vi "Insert_Fix Node Terminals.vi"(6 "Inserted Node":refnum<vi>, 8 "error in (no error)":errorcluster, 9 "Original Wire":refnum<vi>, 11 "Node Name":string) -> (0 "error out":errorcluster)   [LabVIEW 2020]
doc: "When the LabVIEW Insert algorithm inserts the node in a non-ideal manner on a wire, this VI will fix the wiring in those specific cases."
uses:
  <vilib>/Utility/Data Type/Type Definitions/Data Type.ctl
  <vilib>/Utility/Data Type/NI_Data Type.lvlib
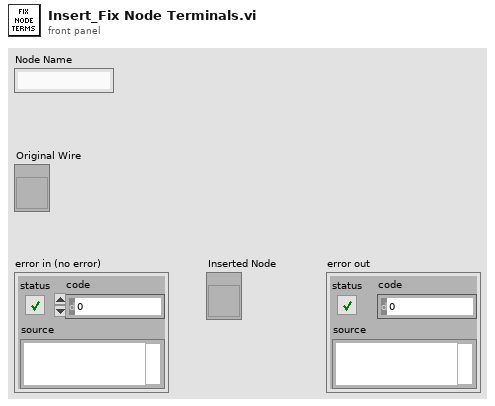
[diagram p1: front panel]
types:
  T1 = typedef "NI_Data Type.lvlib/Data Type.ctl" = enum8{"Invalid Type", "Void", "I8", "I16", "I32", "I64", "U8", "U16", "U32", "U64", "Single Float", "Double Float", "Extended Float", "Single Complex", "Double Complex", "Extended Complex", "Enum U8", "Enum U16", "Enum U32", "Enum U64", "Single Float With Unit", "Double Float With Unit", "Extended Float With Unit", "Single Complex with Unit", "Double Complex with Unit", "Extended Complex with Unit", "Boolean", "String", "Path", "Picture", "Tag", "Array", "Cluster", "Variant", "LV Variant", "Waveform", "Timestamp", "Digital Waveform", "Digital Data", "ExpressData", "Refnum", "External Data", "VI", "Poly VI", "LabVIEW Class Instance", "Fixed Point", "Set Collection", "Map Collection"}
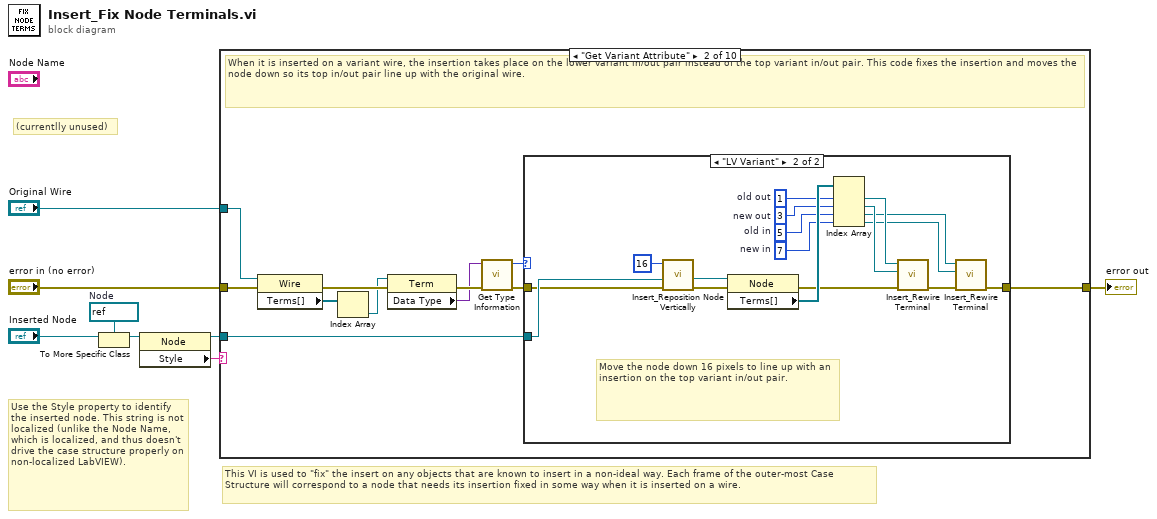
[diagram p0: block diagram]
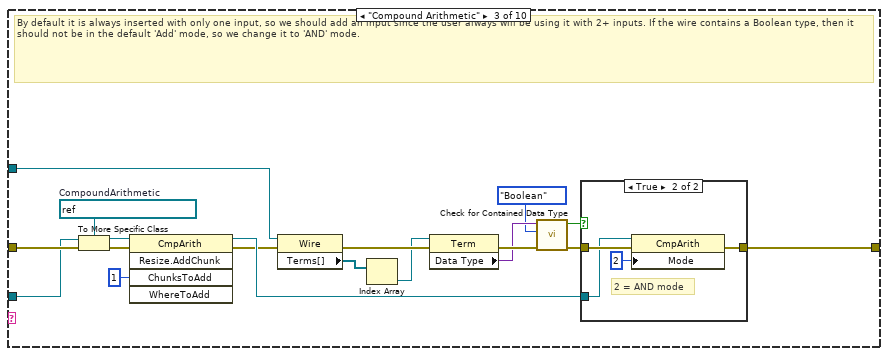
[diagram p4: hidden frame]
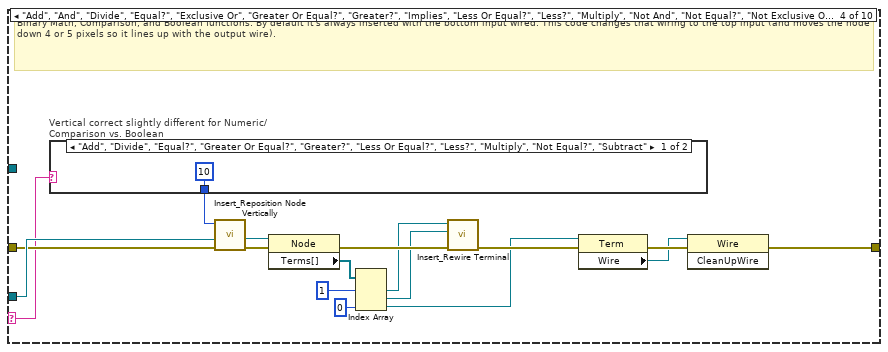
[diagram p6: hidden frame]
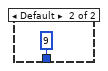
[diagram p7: hidden frame]
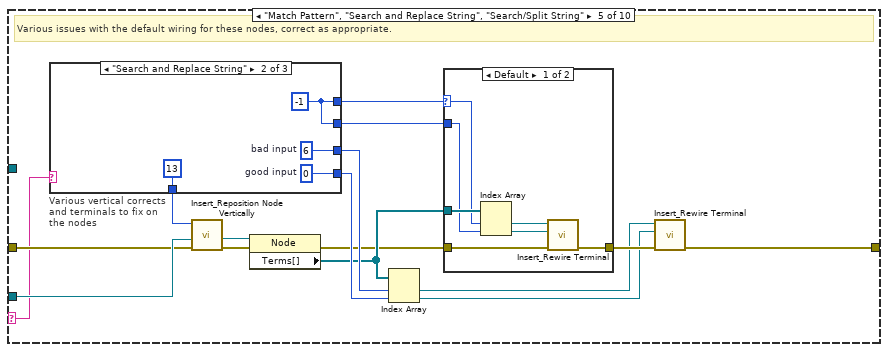
[diagram p8: hidden frame]
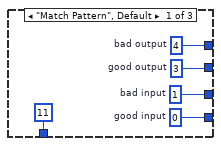
[diagram p10: hidden frame]
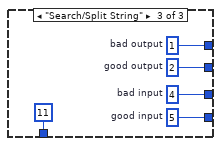
[diagram p11: hidden frame]
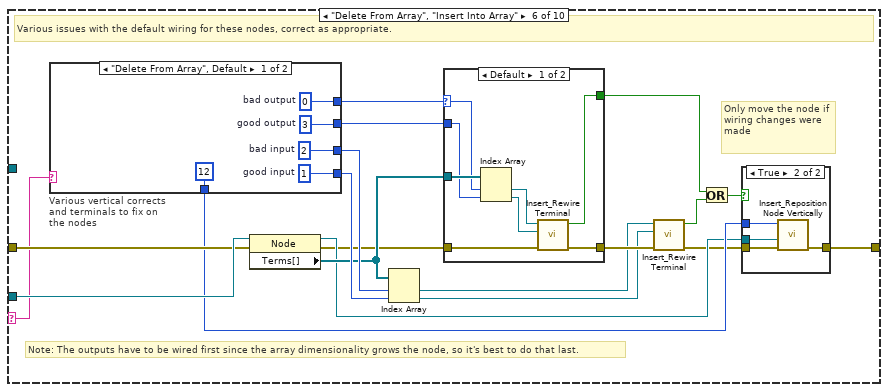
[diagram p12: hidden frame]
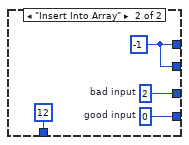
[diagram p15: hidden frame]
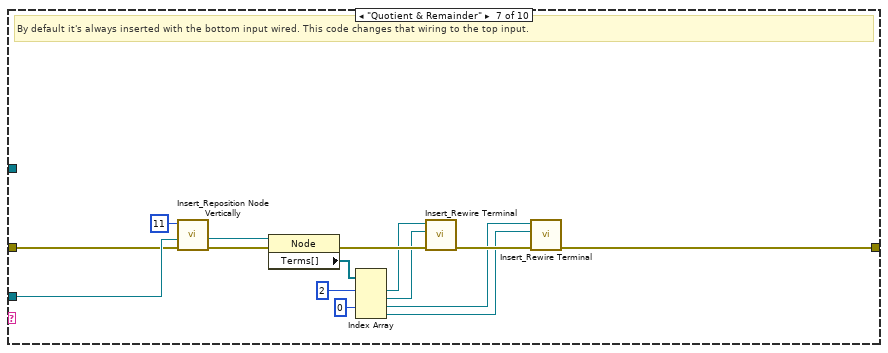
[diagram p16: hidden frame]
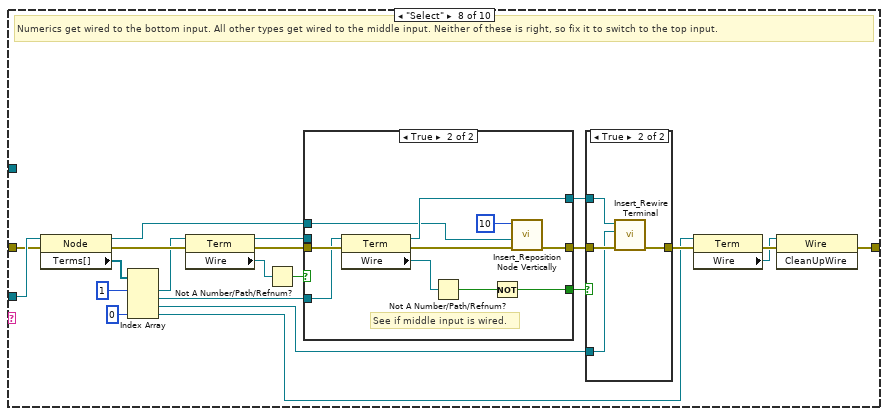
[diagram p17: hidden frame]
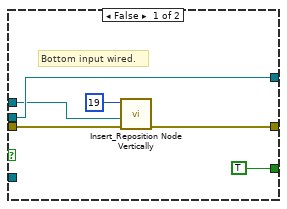
[diagram p19: hidden frame]
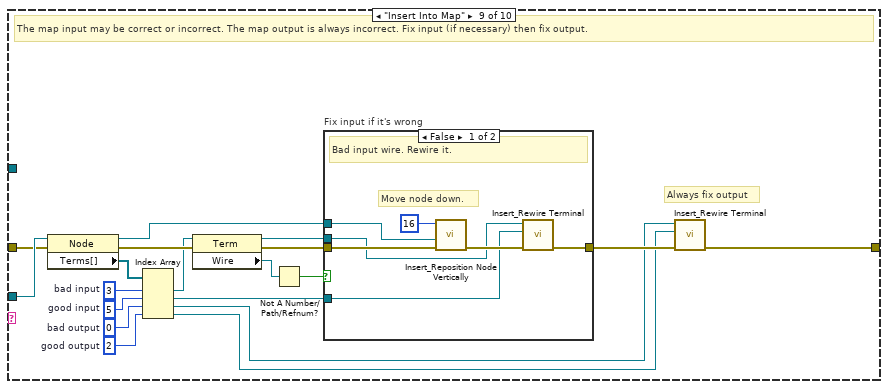
[diagram p20: hidden frame]
diagram:
  w3 = refnum<vi> refnum  # Node
  # "(currentlly unused)"
  # "Use the Style property to identify the inserted node. This string is not localized (unlike the Node Name, which is localized, and thus doesn't drive the case structure properly on non-localized LabVIEW)."
  # "This VI is used to \"fix\" the insert on any objects that are known to insert in a non-ideal way. Each frame of the outer-most Case Structure will correspond to a node that needs its insertion fixed in some way when it is inserted on a wire."
  n1 = To More Specific Class(target class=w3, reference="Inserted Node") -> (specific class reference=w4:refnum<vi>)  [unwired: 1 in, 1 out]
  n2 = property class="Node"(reference=w4) -> (reference out=w2:refnum<vi>, "Style"=w1:string)  [unwired: 1 in, 1 out]
  n3 = case shown="\"Get Variant Attribute\"" w1 {
    selector: w1 -> [_ _ _ w62 w81 w119 _ _ _ _]
    tunnel: "error in (no error)" -> [w9 w20 w44 w77 w95 w136 w174 w196 w236 w263]
    tunnel: [w9 w11 w49 w63 w84 w130 w167 w178 w223 w250] -> w6
    tunnel: "Original Wire" -> [_ w19 w56 _ _ _ _ _ _ _]
    tunnel: w2 -> [_ w10 w43 w78 w96 w137 w175 w197 w237 w264]
    frame Default {
      # "Not a Node that requires wire fixing."
    }
    frame "Get Variant Attribute" {
      # "When it is inserted on a variant wire, the insertion takes place on the lower variant in/out pair instead of the top variant in/out pair. This code fixes the insertion and moves the node down so its top in/out pair line up with the original wire."
      n4 = property class="Wire"(reference=w19, error in=w20) -> (error out=w17:errorcluster, "Terms[]"=w18:refnum<vi>[])  [unwired: 1 out]
      n5 = Index Array(array=w18) -> (element=w16:refnum<vi>)  [unwired: 1 in]
      n6 = property class="Term"(reference=w16, error in=w17) -> (error out=w15:errorcluster, "Data Type"=w14:variant)  [unwired: 1 out]
      n7 = call <vilib>:"Get Type Information.vi"("error in (no error)"=w15, "variant"=w14) -> ("error out"=w13:errorcluster, "type"=w12:T1)  [unwired: 5 in, 3 out]
      n8 = case shown="\"LV Variant\"" w12 {
        tunnel: w13 -> [w21 w37]
        tunnel: [w21 w24] -> w11
        tunnel: w10 -> [_ w38]
        frame Default {
          # "Do nothing if the insert took place on a non-variant wire, like the error cluster."
        }
        frame "LV Variant" {
          w32 = 7  # new in
          w33 = 5  # old in
          w34 = 3  # new out
          w35 = 1  # old out
          # "Move the node down 16 pixels to line up with an insertion on the top variant in/out pair."
          n9 = call <vilib>:"Insert_Reposition Node Vertically.vi"("error in"=w37, "Node in"=w38, "Vertical Change"=16 ("y")) -> ("error out"=w31:errorcluster, "Node out"=w23:refnum<vi>)  [unwired: 7 in]
          n10 = property class="Node"(reference=w23, error in=w31) -> (error out=w30:errorcluster, "Terms[]"=w36:refnum<vi>[])  [unwired: 1 out]
          n11 = Index Array(array=w36, index #1=w35, index #2=w34, index #3=w33, index #4=w32) -> (element #1=w29:refnum<vi>, element #2=w28:refnum<vi>, element #3=w26:refnum<vi>, element #4=w25:refnum<vi>)
          n12 = call <vilib>:"Insert_Rewire Terminal.vi"("error in"=w30, "New Terminal"=w28, "Old Terminal"=w29) -> ("error out"=w27:errorcluster)  [unwired: 7 in, 1 out]
          n13 = call <vilib>:"Insert_Rewire Terminal.vi"("error in"=w27, "New Terminal"=w25, "Old Terminal"=w26) -> ("error out"=w24:errorcluster)  [unwired: 7 in, 1 out]
        }
      }
    }
    frame "Compound Arithmetic" {
      w45 = refnum<vi> refnum  # CompoundArithmetic
      # "By default it is always inserted with only one input, so we should add an input since the user always will be using it with 2+ inputs. If the wire contains a Boolean type, then it should not be in the default 'Add' mode, so we change it to 'AND' mode."
      n14 = To More Specific Class(target class=w45, reference=w43, error in=w44) -> (specific class reference=w47:refnum<vi>, error out=w46:errorcluster)
      n15 = invoke class="CmpArith" method="Resize.AddChunk"(reference=w47, error in=w46, "ChunksToAdd"=u8 1 ("Chunks To Add")) -> (reference out=w42:refnum<vi>, error out=w41:errorcluster)  [unwired: 2 in, 3 out]
      n16 = property class="Wire"(reference=w56, error in=w41) -> (error out=w54:errorcluster, "Terms[]"=w55:refnum<vi>[])  [unwired: 1 out]
      n17 = Index Array(array=w55) -> (element=w53:refnum<vi>)  [unwired: 1 in]
      n18 = property class="Term"(reference=w53, error in=w54) -> (error out=w52:errorcluster, "Data Type"=w51:variant)  [unwired: 1 out]
      n19 = call <vilib>:"Check for Contained Data Type.vi"("error in (no error)"=w52, "data type to find"=Data_Type."Boolean" ("Data Type to Find"), "variant"=w51) -> ("error out"=w50:errorcluster, "contains data type to find?"=w40:bool)  [unwired: 7 in]
      n20 = case shown="True" w40 {
        tunnel: w50 -> [w57 w59]
        tunnel: [w57 w60] -> w49
        tunnel: w42 -> [_ w58]
        frame False {
          # "Wire doesn't contain Boolean, so it's safe to leave CA in 'Add' mode."
        }
        frame True {
          # "2 = AND mode"
          n21 = property class="CmpArith"(reference=w58, error in=w59, "Mode"=u32 2) -> (error out=w60:errorcluster)  [unwired: 1 out]
        }
      }
    }
    frame "Add", "And", "Divide", "Equal?", "Exclusive Or", "Greater Or Equal?", "Greater?", "Implies", "Less Or Equal?", "Less?", "Multiply", "Not And", "Not Equal?", "Not Exclusive Or", "Not Or", "Or", "Subtract" {
      # "Binary Math, Comparison, and Boolean functions: By default it's always inserted with the bottom input wired. This code changes that wiring to the top input (and moves the node down 4 or 5 pixels so it lines up with the output wire)."
      n22 = case "Vertical correct slightly different for Numeric/Comparison vs. Boolean" shown="\"Add\", \"Divide\", \"Equal?\", \"Greater Or Equal?\", \"Greater?\", \"Less Or Equal?\", \"Less?\", \"Multiply\", \"Not Equal?\", \"Subtract\"" w62 {
        tunnel: [10 ("y") 9 ("y")] -> w70
        frame "Add", "Divide", "Equal?", "Greater Or Equal?", "Greater?", "Less Or Equal?", "Less?", "Multiply", "Not Equal?", "Subtract" {
        }
        frame Default {
        }
      }
      n23 = call <vilib>:"Insert_Reposition Node Vertically.vi"("error in"=w77, "Node in"=w78, "Vertical Change"=w70) -> ("error out"=w74:errorcluster, "Node out"=w69:refnum<vi>)  [unwired: 7 in]
      n24 = property class="Node"(reference=w69, error in=w74) -> (error out=w73:errorcluster, "Terms[]"=w76:refnum<vi>[])  [unwired: 1 out]
      n25 = Index Array(array=w76, index #1=1 ("index"), index #3=0 ("index")) -> (element #1=w72:refnum<vi>, element #2=w71:refnum<vi>, element #3=w66:refnum<vi>)  [unwired: 1 in]
      n26 = call <vilib>:"Insert_Rewire Terminal.vi"("error in"=w73, "New Terminal"=w71, "Old Terminal"=w72) -> ("error out"=w67:errorcluster)  [unwired: 7 in, 1 out]
      n27 = property class="Term"(reference=w66, error in=w67) -> (error out=w65:errorcluster, "Wire"=w64:refnum<vi>)  [unwired: 1 out]
      n28 = invoke class="Wire" method="CleanUpWire"(reference=w64, error in=w65) -> (error out=w63:errorcluster)  [unwired: 1 in, 2 out]
    }
    frame "Match Pattern", "Search and Replace String", "Search/Split String" {
      # "Various issues with the default wiring for these nodes, correct as appropriate."
      n29 = case "Various vertical corrects and terminals to fix on the nodes" shown="\"Search and Replace String\"" w81 {
        tunnel: [11 ("y") 13 ("y") 11 ("y")] -> w82
        tunnel: [w108 w112 w117] -> w94
        tunnel: [w107 w111 w116] -> w93
        tunnel: [w106 w110 w115] -> w92
        tunnel: [w105 w110 w114] -> w91
        frame "Match Pattern", Default {
          w105 = 3  # good output
          w106 = 4  # bad output
          w107 = 0  # good input
          w108 = 1  # bad input
        }
        frame "Search and Replace String" {
          w110 = -1 ("bad output")
          w111 = 0  # good input
          w112 = 6  # bad input
        }
        frame "Search/Split String" {
          w114 = 2  # good output
          w115 = 1  # bad output
          w116 = 5  # good input
          w117 = 4  # bad input
        }
      }
      n30 = call <vilib>:"Insert_Reposition Node Vertically.vi"("error in"=w95, "Node in"=w96, "Vertical Change"=w82) -> ("error out"=w88:errorcluster, "Node out"=w83:refnum<vi>)  [unwired: 7 in]
      n31 = property class="Node"(reference=w83, error in=w88) -> (error out=w89:errorcluster, "Terms[]"=w90:refnum<vi>[])  [unwired: 1 out]
      n32 = Index Array(array=w90, index #1=w94, index #2=w93) -> (element #1=w86:refnum<vi>, element #2=w85:refnum<vi>)
      n33 = case shown="Default" w92 {
        selector: w92 -> [w101 _]
        tunnel: w89 -> [w100 w104]
        tunnel: [w97 w104] -> w87
        tunnel: w91 -> [w102 _]
        tunnel: w90 -> [w103 _]
        frame Default {
          n34 = Index Array(array=w103, index #1=w101, index #2=w102) -> (element #1=w99:refnum<vi>, element #2=w98:refnum<vi>)
          n35 = call <vilib>:"Insert_Rewire Terminal.vi"("error in"=w100, "New Terminal"=w98, "Old Terminal"=w99) -> ("error out"=w97:errorcluster)  [unwired: 7 in, 1 out]
        }
        frame -1 {
          # "No output fix required."
        }
      }
      n36 = call <vilib>:"Insert_Rewire Terminal.vi"("error in"=w87, "New Terminal"=w85, "Old Terminal"=w86) -> ("error out"=w84:errorcluster)  [unwired: 7 in, 1 out]
    }
    frame "Delete From Array", "Insert Into Array" {
      # "Only move the node if wiring changes were made"
      # "Note: The outputs have to be wired first since the array dimensionality grows the node, so it's best to do that last."
      # "Various issues with the default wiring for these nodes, correct as appropriate."
      n37 = case "Various vertical corrects and terminals to fix on the nodes" shown="\"Delete From Array\", Default" w119 {
        tunnel: [12 ("y") 12 ("y")] -> w127
        tunnel: [w155 w159] -> w135
        tunnel: [w154 w158] -> w134
        tunnel: [w153 w157] -> w133
        tunnel: [w152 w157] -> w132
        frame "Delete From Array", Default {
          w152 = 3  # good output
          w153 = 0  # bad output
          w154 = 1  # good input
          w155 = 2  # bad input
        }
        frame "Insert Into Array" {
          w157 = -1 ("bad output")
          w158 = 0  # good input
          w159 = 2  # bad input
        }
      }
      n38 = property class="Node"(reference=w137, error in=w136) -> (reference out=w126:refnum<vi>, error out=w125:errorcluster, "Terms[]"=w131:refnum<vi>[])
      n39 = Index Array(array=w131, index #1=w135, index #2=w134) -> (element #1=w122:refnum<vi>, element #2=w121:refnum<vi>)
      n40 = case shown="Default" w133 {
        selector: w133 -> [w147 _]
        tunnel: w125 -> [w145 w151]
        tunnel: [w150 w151] -> w124
        tunnel: w132 -> [w148 _]
        tunnel: w131 -> [w149 _]
        tunnel: [w143 _] -> w129
        frame Default {
          n41 = Index Array(array=w149, index #1=w147, index #2=w148) -> (element #1=w144:refnum<vi>, element #2=w146:refnum<vi>)
          n42 = call <vilib>:"Insert_Rewire Terminal.vi"("error in"=w145, "New Terminal"=w146, "Old Terminal"=w144) -> ("error out"=w150:errorcluster, "Terminals Rewired?"=w143:bool)  [unwired: 7 in]
        }
        frame -1 {
          # "No output fix required."
        }
      }
      n43 = call <vilib>:"Insert_Rewire Terminal.vi"("error in"=w124, "New Terminal"=w121, "Old Terminal"=w122) -> ("error out"=w123:errorcluster, "Terminals Rewired?"=w120:bool)  [unwired: 7 in]
      n44 = Or(x=w129, y=w120) -> (x .or. y?=w128:bool)
      n45 = case shown="True" w128 {
        tunnel: w123 -> [w138 w142]
        tunnel: [w138 w141] -> w130
        tunnel: w127 -> [_ w140]
        tunnel: w126 -> [_ w139]
        frame False {
        }
        frame True {
          n46 = call <vilib>:"Insert_Reposition Node Vertically.vi"("error in"=w142, "Node in"=w139, "Vertical Change"=w140) -> ("error out"=w141:errorcluster)  [unwired: 7 in, 1 out]
        }
      }
    }
    frame "Quotient & Remainder" {
      # "By default it's always inserted with the bottom input wired. This code changes that wiring to the top input."
      n47 = call <vilib>:"Insert_Reposition Node Vertically.vi"("error in"=w174, "Node in"=w175, "Vertical Change"=11) -> ("error out"=w163:errorcluster, "Node out"=w162:refnum<vi>)  [unwired: 7 in]
      n48 = property class="Node"(reference=w162, error in=w163) -> (error out=w171:errorcluster, "Terms[]"=w173:refnum<vi>[])  [unwired: 1 out]
      n49 = Index Array(array=w173, index #1=2 ("index"), index #3=0 ("index")) -> (element #1=w170:refnum<vi>, element #2=w169:refnum<vi>, element #3=w165:refnum<vi>, element #4=w164:refnum<vi>)  [unwired: 2 in]
      n50 = call <vilib>:"Insert_Rewire Terminal.vi"("error in"=w171, "New Terminal"=w169, "Old Terminal"=w170) -> ("error out"=w168:errorcluster)  [unwired: 7 in, 1 out]
      n51 = call <vilib>:"Insert_Rewire Terminal.vi"("error in"=w168, "New Terminal"=w164, "Old Terminal"=w165) -> ("error out"=w167:errorcluster)  [unwired: 7 in, 1 out]
    }
    frame "Select" {
      # "Numerics get wired to the bottom input. All other types get wired to the middle input. Neither of these is right, so fix it to switch to the top input."
      n52 = property class="Node"(reference=w197, error in=w196) -> (reference out=w186:refnum<vi>, error out=w193:errorcluster, "Terms[]"=w195:refnum<vi>[])
      n53 = Index Array(array=w195, index #1=1 ("index"), index #4=0 ("index")) -> (element #1=w192:refnum<vi>, element #2=w188:refnum<vi>, element #3=w182:refnum<vi>, element #4=w177:refnum<vi>)  [unwired: 2 in]
      n54 = property class="Term"(reference=w192, error in=w193) -> (reference out=w190:refnum<vi>, error out=w189:errorcluster, "Wire"=w183:refnum<vi>)
      n55 = Not A Number/Path/Refnum?(number/path/refnum=w183) -> (NaN/Path/Refnum?=w191:bool)
      n56 = case shown="True" w191 {
        tunnel: w190 -> [w208 _]
        tunnel: w189 -> [w206 w218]
        tunnel: w188 -> [_ w217]
        tunnel: [w205 w210] -> w187
        tunnel: w186 -> [w203 w209]
        tunnel: [w208 w214] -> w185
        tunnel: [TRUE w213] -> w184
        frame False {
          # "Bottom input wired."
          n57 = call <vilib>:"Insert_Reposition Node Vertically.vi"("error in"=w206, "Node in"=w203, "Vertical Change"=19 ("y")) -> ("error out"=w205:errorcluster)  [unwired: 7 in, 1 out]
        }
        frame True {
          # "See if middle input is wired."
          n58 = property class="Term"(reference=w217, error in=w218) -> (reference out=w214:refnum<vi>, error out=w211:errorcluster, "Wire"=w216:refnum<vi>)
          n59 = Not A Number/Path/Refnum?(number/path/refnum=w216) -> (NaN/Path/Refnum?=w215:bool)
          n60 = Not(x=w215) -> (.not. x?=w213:bool)
          n61 = call <vilib>:"Insert_Reposition Node Vertically.vi"("error in"=w211, "Node in"=w209, "Vertical Change"=10 ("y")) -> ("error out"=w210:errorcluster)  [unwired: 7 in, 1 out]
        }
      }
      n62 = case shown="True" w184 {
        tunnel: [w198 w199] -> w180
        tunnel: w182 -> [_ w200]
        tunnel: w187 -> [w198 w202]
        tunnel: w185 -> [_ w201]
        frame False {
          # "Unknown wiring pattern. Don't do anything."
        }
        frame True {
          n63 = call <vilib>:"Insert_Rewire Terminal.vi"("error in"=w202, "New Terminal"=w200, "Old Terminal"=w201) -> ("error out"=w199:errorcluster)  [unwired: 7 in, 1 out]
        }
      }
      n64 = property class="Term"(reference=w177, error in=w180) -> (error out=w179:errorcluster, "Wire"=w176:refnum<vi>)  [unwired: 1 out]
      n65 = invoke class="Wire" method="CleanUpWire"(reference=w176, error in=w179) -> (error out=w178:errorcluster)  [unwired: 1 in, 2 out]
    }
    frame "Insert Into Map" {
      w221 = 2  # good output
      w222 = 0  # bad output
      w224 = 5  # good input
      w234 = 3  # bad input
      # "Always fix output"
      # "The map input may be correct or incorrect. The map output is always incorrect. Fix input (if necessary) then fix output."
      n66 = property class="Node"(reference=w237, error in=w236) -> (reference out=w226:refnum<vi>, error out=w233:errorcluster, "Terms[]"=w235:refnum<vi>[])
      n67 = Index Array(array=w235, index #1=w234, index #2=w224, index #3=w222, index #4=w221) -> (element #1=w232:refnum<vi>, element #2=w228:refnum<vi>, element #3=w219:refnum<vi>, element #4=w220:refnum<vi>)
      n68 = property class="Term"(reference=w232, error in=w233) -> (reference out=w230:refnum<vi>, error out=w229:errorcluster, "Wire"=w225:refnum<vi>)
      n69 = Not A Number/Path/Refnum?(number/path/refnum=w225) -> (NaN/Path/Refnum?=w231:bool)
      n70 = case "Fix input if it's wrong" shown="False" w231 {
        tunnel: w230 -> [w239 _]
        tunnel: w229 -> [w244 w245]
        tunnel: w228 -> [w238 _]
        tunnel: [w240 w245] -> w227
        tunnel: w226 -> [w242 _]
        frame False {
          # "Move node down."
          # "Bad input wire. Rewire it."
          n71 = call <vilib>:"Insert_Reposition Node Vertically.vi"("error in"=w244, "Node in"=w242, "Vertical Change"=16 ("y")) -> ("error out"=w241:errorcluster)  [unwired: 7 in, 1 out]
          n72 = call <vilib>:"Insert_Rewire Terminal.vi"("error in"=w241, "New Terminal"=w238, "Old Terminal"=w239) -> ("error out"=w240:errorcluster)  [unwired: 7 in, 1 out]
        }
        frame True {
          # "Input wire is already good."
        }
      }
      n73 = call <vilib>:"Insert_Rewire Terminal.vi"("error in"=w227, "New Terminal"=w220, "Old Terminal"=w219) -> ("error out"=w223:errorcluster)  [unwired: 7 in, 1 out]
    }
    frame "Insert Into Set" {
      w248 = 1  # good output
      w249 = 0  # bad output
      w251 = 3  # good input
      w261 = 2  # bad input
      # "Always fix output"
      # "The set input and output may be correct or incorrect, depending on the data type of the set."
      n74 = property class="Node"(reference=w264, error in=w263) -> (reference out=w253:refnum<vi>, error out=w260:errorcluster, "Terms[]"=w262:refnum<vi>[])
      n75 = Index Array(array=w262, index #1=w261, index #2=w251, index #3=w249, index #4=w248) -> (element #1=w259:refnum<vi>, element #2=w255:refnum<vi>, element #3=w246:refnum<vi>, element #4=w247:refnum<vi>)
      n76 = property class="Term"(reference=w259, error in=w260) -> (reference out=w257:refnum<vi>, error out=w256:errorcluster, "Wire"=w252:refnum<vi>)
      n77 = Not A Number/Path/Refnum?(number/path/refnum=w252) -> (NaN/Path/Refnum?=w258:bool)
      n78 = case "Fix input if it's wrong" shown="False" w258 {
        tunnel: w257 -> [w266 _]
        tunnel: w256 -> [w271 w272]
        tunnel: w255 -> [w265 _]
        tunnel: [w267 w272] -> w254
        tunnel: w253 -> [w269 _]
        frame False {
          # "Move node down."
          # "Bad input wire. Rewire it."
          n79 = call <vilib>:"Insert_Reposition Node Vertically.vi"("error in"=w271, "Node in"=w269, "Vertical Change"=8 ("y")) -> ("error out"=w268:errorcluster)  [unwired: 7 in, 1 out]
          n80 = call <vilib>:"Insert_Rewire Terminal.vi"("error in"=w268, "New Terminal"=w265, "Old Terminal"=w266) -> ("error out"=w267:errorcluster)  [unwired: 7 in, 1 out]
        }
        frame True {
          # "Input wire is already good."
        }
      }
      n81 = call <vilib>:"Insert_Rewire Terminal.vi"("error in"=w254, "New Terminal"=w247, "Old Terminal"=w246) -> ("error out"=w250:errorcluster)  [unwired: 7 in, 1 out]
    }
  }
  "error out" <- w6
